vi "Add Target Reply Protocol.vi"(8 "error in":errorcluster, 11 "Reply Protocol Manager in":refnum<class "Reply Protocol Manager.lvclass">) -> (0 "error out":errorcluster)   [LabVIEW 2023, in "HAL GOOP4.lvlib" / "Measure and Stimulus Subsystems.lvclass"]
uses:
  Measure and Stimulus Subsystems.lvclass
  Measure and Stimulus Subsystems.lvclass/Measure and Stimulus Subsystems.ctl
  Reply Protocol Manager/Reply Protocol Manager.lvclass
  Reply Protocol/Reply Protocol Base/Reply Protocol Base.lvclass
panel:
  out "Reply Protocol Manager out":refnum<class "Reply Protocol Manager.lvclass">
  in  "Reply Protocol Base":refnum<class "Reply Protocol Base.lvclass">
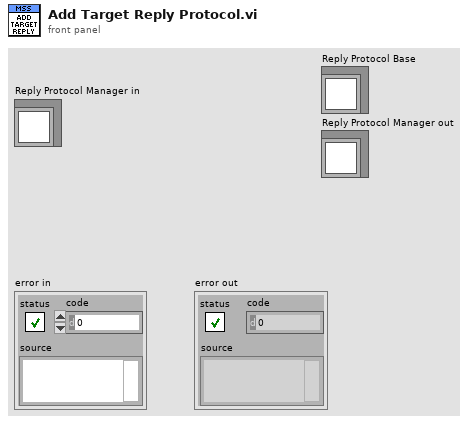
[diagram p1: front panel]
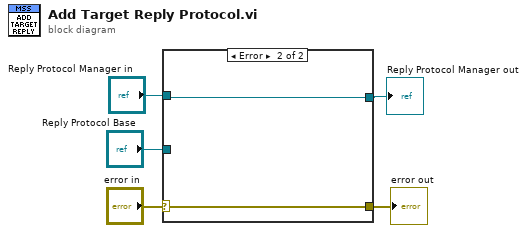
[diagram p0: block diagram]
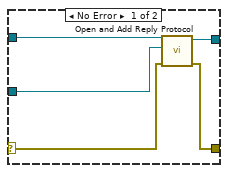
[diagram p2: hidden frame]
diagram:
  n1 = case shown="Error" "error in" {
    selector: "error in" -> [w8 w12]
    tunnel: [w9 w12] -> w4
    tunnel: "Reply Protocol Manager in" -> [w10 w11]
    tunnel: "Reply Protocol Base" -> [w7 _]
    tunnel: [w6 w11] -> w1
    frame No Error {
      n2 = call "Open and Add Reply Protocol.vi"("Error In"=w8, "Reply Protocol Base"=w7, "reference in"=w10) -> ("Error Out"=w9:errorcluster, "reference out"=w6:refnum<class "Reply Protocol Manager.lvclass">)  [unwired: 7 in]
    }
    frame Error {
    }
  }
  "error out" <- w4
  "Reply Protocol Manager out" <- w1
